vi "Furnace PID SP 2.vi"(6 "PID gains":T1={"proportional gain (Kc)"=1.0, "integral time (Ti, min)"=0.1, "derivative time (Td, min)"=0.0}, 10 "PV deg C":dbl format="%.2f", 11 "User SP Deg C":dbl format="%.2f") -> (2 "output T SP":dbl format="%.2f")   [LabVIEW 2014]
uses:
  <vilib>/addons/control/pid/pid.llb/PID (DBL).vi
  <vilib>/addons/control/pid/NI_PID_pid.lvlib
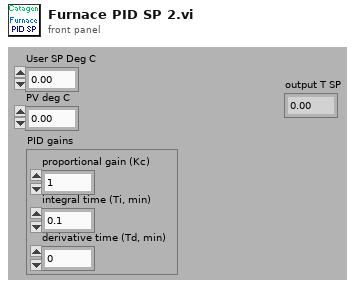
[diagram p1: front panel]
types:
  T1 = cluster{"proportional gain (Kc)":dbl, "integral time (Ti, min)":dbl, "derivative time (Td, min)":dbl}
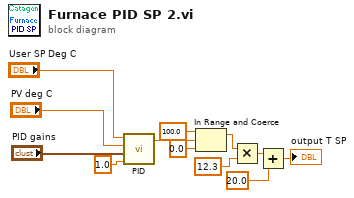
[diagram p0: block diagram]
diagram:
  n1 = call-poly <vilib>:"PID.vi"("dt (s)"=1.0, "PID gains"="PID gains", "process variable"="PV deg C", "setpoint"="User SP Deg C") -> ("output"=w9:dbl)  [unwired: 6 in, 1 out]
  n2 = In Range and Coerce(upper limit=100.0, x=w9, lower limit=0.0) -> (coerced(x)=w5:dbl)  [unwired: 1 out]
  n3 = Multiply(x=w5, y=12.3) -> (x*y=w3:dbl)
  n4 = Add(x=w3, y=20.0) -> (x+y=→"output T SP":dbl)
